vi "CheckSN.vi"(6 "Slot":T1, 8 "error out":errorcluster, 11 "SN":string) -> (0 "错误输出":errorcluster, 3 "比对结果":bool)   [LabVIEW 2013]
uses:
  SystemCode/SysControl/Slot.ctl
panel:
  out "提示":string
  out "当前SN":string
  in  "扫描SN":string
  in  "停止":bool
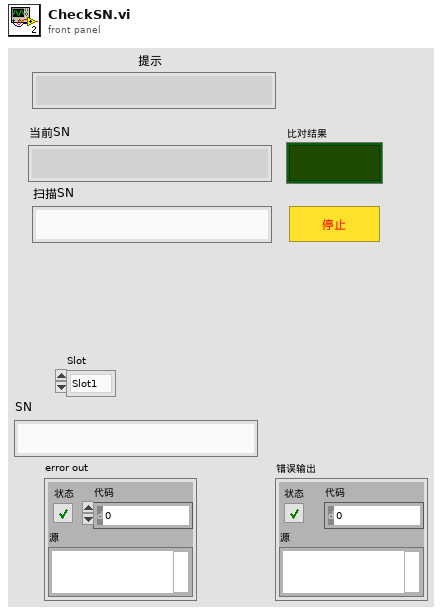
[diagram p1: front panel]
types:
  T1 = typedef "Slot.ctl" = enum16{"Slot1", "Slot2", "Slot3", "Slot4"}
  T2 = typedef "LVRectTypeDef.ctl" = cluster{"Left":i16, "Top":i16, "Right":i16, "Bottom":i16}
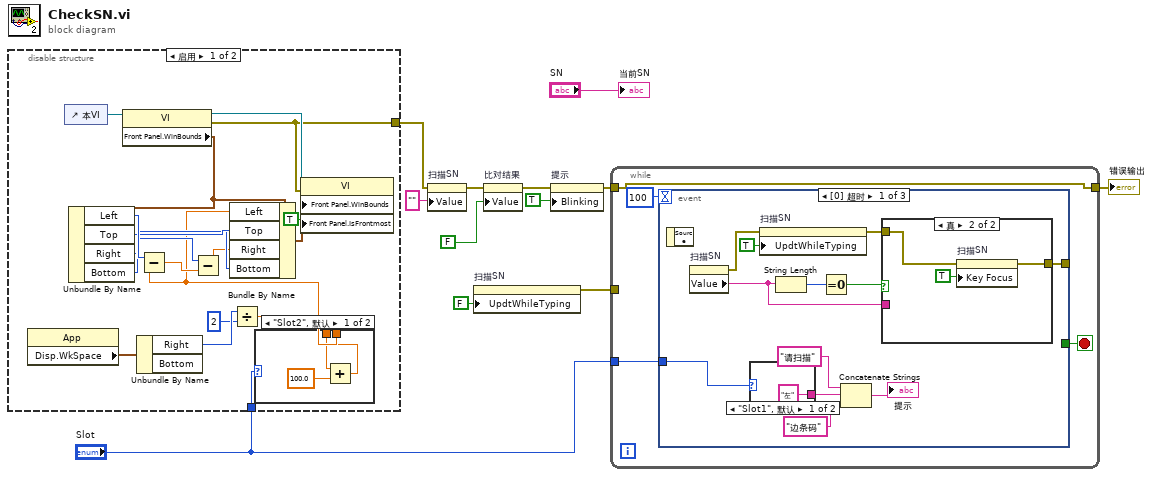
[diagram p0: block diagram]
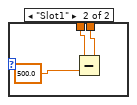
[diagram p2: hidden frame]
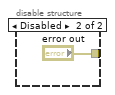
[diagram p3: hidden frame]
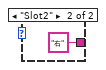
[diagram p4: hidden frame]
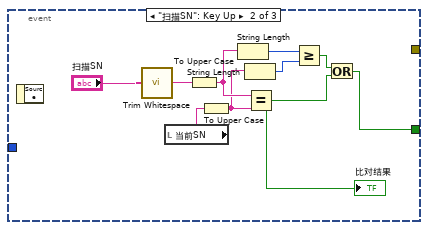
[diagram p6: hidden frame]
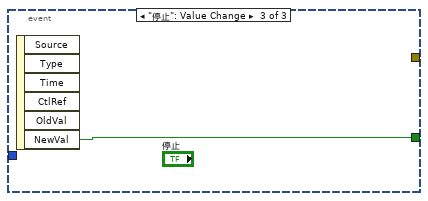
[diagram p7: hidden frame]
diagram:
  n1 = disable-structure shown="启用" {
    disable-tunnel: [w18 "error out"] -> w12
    disable-tunnel: "Slot" -> [w13 _]
    frame Enabled {
      n2 = property class="App"() -> ("Disp.WkSpace"=w27:T2)  [unwired: 2 in, 2 out]
      n3 = control-ref of="本VI"() -> (w30:refnum<vi>)
      n4 = property class="VI"(reference=w30) -> (reference out=w29:refnum<vi>, error out=w18:errorcluster, "Front Panel.WinBounds"=w25:T2)  [unwired: 1 in]
      n5 = Unbundle By Name(w25) -> ("Left"=w24:i16, "Top"=w23:i16, "Right"=w21:i16, "Bottom"=w22:i16)
      n6 = Unbundle By Name(w27) -> ("Right"=w17:i16)  [unwired: 1 out]
      n7 = Divide(x=w17, y=i16 2) -> (x/y=w15:dbl)
      n8 = case shown="\"Slot2\", 默认" w13 {
        tunnel: w15 -> [w33 w36]
        tunnel: [w31 w34] -> w14
        frame "Slot2", Default {
          n9 = Add(x=w33, y=100.0) -> (x+y=w31:dbl)
        }
        frame "Slot1" {
          n10 = Subtract(x=w36, y=500.0) -> (x-y=w34:dbl)
        }
      }
      n11 = Subtract(x=w24, y=w14) -> (x-y=w20:dbl)
      n12 = Subtract(x=w21, y=w20) -> (x-y=w19:dbl)
      n13 = Bundle By Name(cluster=w25, "Left"=w14, "Top"=w23, "Right"=w19, "Bottom"=w22) -> (w28:T2)
      n14 = property class="VI"(reference=w29, error in=w18, "Front Panel.WinBounds"=w28, "Front Panel.IsFrontmost"=TRUE ("前面板窗口:可调整大小")) -> ()  [unwired: 2 out]
    }
    frame Disabled {
    }
  }
  n15 = property on="扫描SN" class="Str"(error in=w12, "Value"="" ("扫描SN")) -> (error out=w8:errorcluster)  [unwired: 1 in, 1 out]
  n16 = property on="扫描SN" class="Str"("UpdtWhileTyping"=FALSE ("键入时刷新？")) -> (error out=w2:errorcluster)  [unwired: 2 in, 1 out]
  n17 = property on="比对结果" class="Bool (严格)"(error in=w8, "Value"=FALSE) -> (error out=w7:errorcluster)  [unwired: 1 in, 1 out]
  n18 = property on="提示" class="Str"(error in=w7, "Blinking"=TRUE ("闪烁")) -> (error out=w10:errorcluster)  [unwired: 1 in, 1 out]
  n19 = while {
    tunnel: w10 -> [w39]
    tunnel: [w39] -> w6
    tunnel: "Slot" -> [w38]
    tunnel: w2 -> [_]
    stop <- w41 stop-if-true
    n20 = event shown="[0] 超时" {
      selector: _ -> [_ _ _]
      dyn-events: _ -> [_ _ _]
      timeout: 100 -> [_ _ _]
      tunnel: [_ w60 w69] -> w41
      tunnel: w38 -> [w49 _ _]
      tunnel: [w42 _ _] -> _
      event Timeout {
        n21 = event-data() -> ()  [unwired: 1 in, 1 out]
        n22 = property on="扫描SN" class="Str"() -> (error out=w45:errorcluster, "Value"=w48:string)  [unwired: 2 in, 1 out]
        n23 = case shown="\"Slot1\", 默认" w49 {
          tunnel: ["左" ("字符串") "右" ("字符串")] -> w50
          frame "Slot1", Default {
          }
          frame "Slot2" {
          }
        }
        n24 = property on="扫描SN" class="Str"(error in=w45, "UpdtWhileTyping"=TRUE ("键入时刷新？")) -> (error out=w43:errorcluster)  [unwired: 1 in, 1 out]
        n25 = String Length(string=w48) -> (length=w46:i32)
        n26 = Equal To 0?(x=w46) -> (x = 0?=w53:bool)
        n27 = Concatenate Strings("请扫描" ("字符串"), w50, "边条码" ("字符串")) -> (→"提示":string)
        n28 = case shown="真" w53 {
          tunnel: w48 -> [_ _]
          tunnel: w43 -> [_ w57]
          tunnel: [_ w56] -> w42
          frame False {
          }
          frame True {
            n29 = property on="扫描SN" class="Str"(error in=w57, "Key Focus"=TRUE ("键选中")) -> (error out=w56:errorcluster)  [unwired: 1 in, 1 out]
          }
        }
      }
      event "扫描SN": Key Up {
        n30 = event-data() -> ()  [unwired: 1 in, 1 out]
        n31 = call <vilib>:"Trim Whitespace.vi"("string"="扫描SN") -> ("trimmed string"=w68:string)  [unwired: 1 in]
        n32 = local read "当前SN"() -> (w67:string)
        n33 = To Upper Case(1:w68) -> (0:w66:string)
        n34 = To Upper Case(1:w67) -> (0:w65:string)
        n35 = String Length(string=w66) -> (length=w64:i32)
        n36 = String Length(string=w65) -> (length=w63:i32)
        n37 = Equal?(x=w66, y=w65) -> (x = y?=w61:bool)
        "比对结果" <- w61
        n38 = Greater Or Equal?(x=w64, y=w63) -> (x >= y?=w62:bool)
        n39 = Or(x=w62, y=w61) -> (x .or. y?=w60:bool)
      }
      event "停止": Value Change {
        n40 = event-data() -> ("NewVal"=w69:bool)  [unwired: 1 in, 5 out]
      }
    }
  }
  "错误输出" <- w6
  "当前SN" <- "SN"
